vi "PH_Tektronix_7000.PC Write PSDB.vi"(0 "i ref in":refnum<vi>, 5 "error IO":errorcluster) -> (14 "i ref out":refnum<vi>, 19 "error out":errorcluster)   [LabVIEW 2014, in "PH_Tektronix_7000.lvlib"]
doc: "This is the proc case which writes data to the PHELIX shot data base."
uses:
  PH_Tektronix_7000.lvlib
  PH_PSDBWriter/PH_PSDBWriter.String dataset.ctl
  PH_PSDBWriter/PH_PSDBWriter.Numeric dataset.ctl
  PH_StatusHandler/PH_StatusHandler.lvlib
  PH_PSDBWriter/PH_PSDBWriter.lvlib
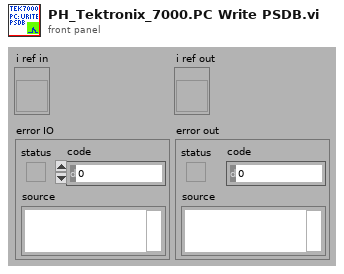
[diagram p1: front panel]
types:
  T1 = typedef "PH_PSDBWriter.lvlib/PH_PSDBWriter.Numeric dataset.ctl" = cluster{"name":string, "data":dbl, "unit":string}
  T2 = typedef "PH_PSDBWriter.lvlib/PH_PSDBWriter.String dataset.ctl" = cluster{"name":string, "data":string, "unit":string}
  T3 = typedef "PH_Tektronix_7000.lvlib/PH_Tektronix_7000.i attribute.ctl" = cluster{"VISA Resource Name":refnum<visa-resource-name>, "IDN":cluster{"Instrument Driver":string, "Instrument Firmware":string, "Model":string, "Serial Number":string}, "Selftest":cluster{"Result":i32, "Message":string}, "Trigger Configuration":T4, "Acquisition Configuration":T5, "GUI Refs":T6, "State":T7, "Error Message":string, "Allow Prdc Loop?":bool, "Channel 1":T8, "Channel 2":T8, "Channel 3":T8, "Channel 4":T8, "Data CH 1":waveform(dbl), "Data CH 2":waveform(dbl), "Data CH 3":waveform(dbl), "Data CH 4":waveform(dbl), "Allow config?":bool, "Name Channel 1":string, "Name Channel 2":string, "Name Channel 3":string, "Name Channel 4":string, "Fetch Data before sending to PSDB?":bool, "Constructor passed?":bool, "Data taken at":timestamp, "Plot Colors":u32[], "Default VISA Resource":string}
  T4 = typedef "PH_Tektronix_7000.lvlib/PH_Tektronix_7000.Trigger Config.ctl" = cluster{"Source":u16, "Level [V]":dbl, "Slope":u16, "Coupling":u16, "Trigger Mode":u16}
  T5 = typedef "PH_Tektronix_7000.lvlib/PH_Tektronix_7000.Acquisition Config.ctl" = cluster{"Record Length":u32, "Timebase [s/div]":dbl, "Position [%]":dbl, "Acquisition Type":u16, "Average Waveforms":i32, "Envelope Waveforms":i32, "WfmDB Samples":i32, "Continuous?":bool, "Delay [s]":dbl, "Run?":bool}
  T6 = typedef "PH_Tektronix_7000.lvlib/PH_Tektronix_7000.GUI Refs.ctl" = cluster{"Graph":refnum<vi>, "State":refnum<vi>, "Delete":refnum<vi>, "VISA Resource":refnum<vi>, "Allow Configure":refnum<vi>, "Fetch Data":refnum<vi>, "Fetch before sending Data to PSDB":refnum<vi>, "Name Channel 1":refnum<vi>, "Name Channel 2":refnum<vi>, "Name Channel 3":refnum<vi>, "Name Channel 4":refnum<vi>, "Prdc Intervall [ms]":refnum<vi>, "Data taken":refnum<vi>, "Model":refnum<vi>, "Serial Number":refnum<vi>, "Firmware":refnum<vi>, "Driver":refnum<vi>, "Acquisition":refnum<vi>, "Trigger":refnum<vi>, "Cursor: D Time [s]":refnum<vi>, "Cursor: D Signal [V]":refnum<vi>, "Channel 1":refnum<vi>, "Channel 2":refnum<vi>, "Channel 3":refnum<vi>, "Channel 4":refnum<vi>}
  T7 = typedef "PH_StatusHandler.lvlib/PH_StatusHandler.Status.ctl" = i16
  T8 = typedef "PH_Tektronix_7000.lvlib/PH_Tektronix_7000.Channel Config.ctl" = cluster{"Enable Channel":bool, "Bandwidth":u16, "Input Impedance":u16, "Vertical Coupling":u16, "Probe Attenuation":dbl, "Range [V/div]":dbl, "Position [div]":dbl, "Bandwidth raw":string}
  T9 = typedef "PH_PSDBWriter.lvlib/PH_PSDBWriter.Boolean dataset.ctl" = cluster{"name":string, "data":bool, "unit":string}
  T10 = typedef "PH_PSDBWriter.lvlib/PH_PSDBWriter.2D dataset.ctl" = cluster{"name":string, "data":dbl[][], "axis description":T11}
  T11 = typedef "PSDB.lvlib/PSDB_AxisDescription.ctl" = cluster{"x axis label":string, "y axis label":string, "x axis unit":string, "y axis unit":string}
  T12 = typedef "PH_PSDBWriter.lvlib/PH_PSDBWriter.PSDB Dataset.ctl" = cluster{"Version":i32, "2D data Input":T10[], "Boolean Input":T9[], "Image Input":T13[], "Numeric Input":T1[], "String Input":T2[]}
  T13 = typedef "PH_PSDBWriter.lvlib/PH_PSDBWriter.Image dataset.ctl" = cluster{"name":string, "data":T14, "unit":string}
  T14 = typedef "IMAQ Image.ctl" = refnum<image>
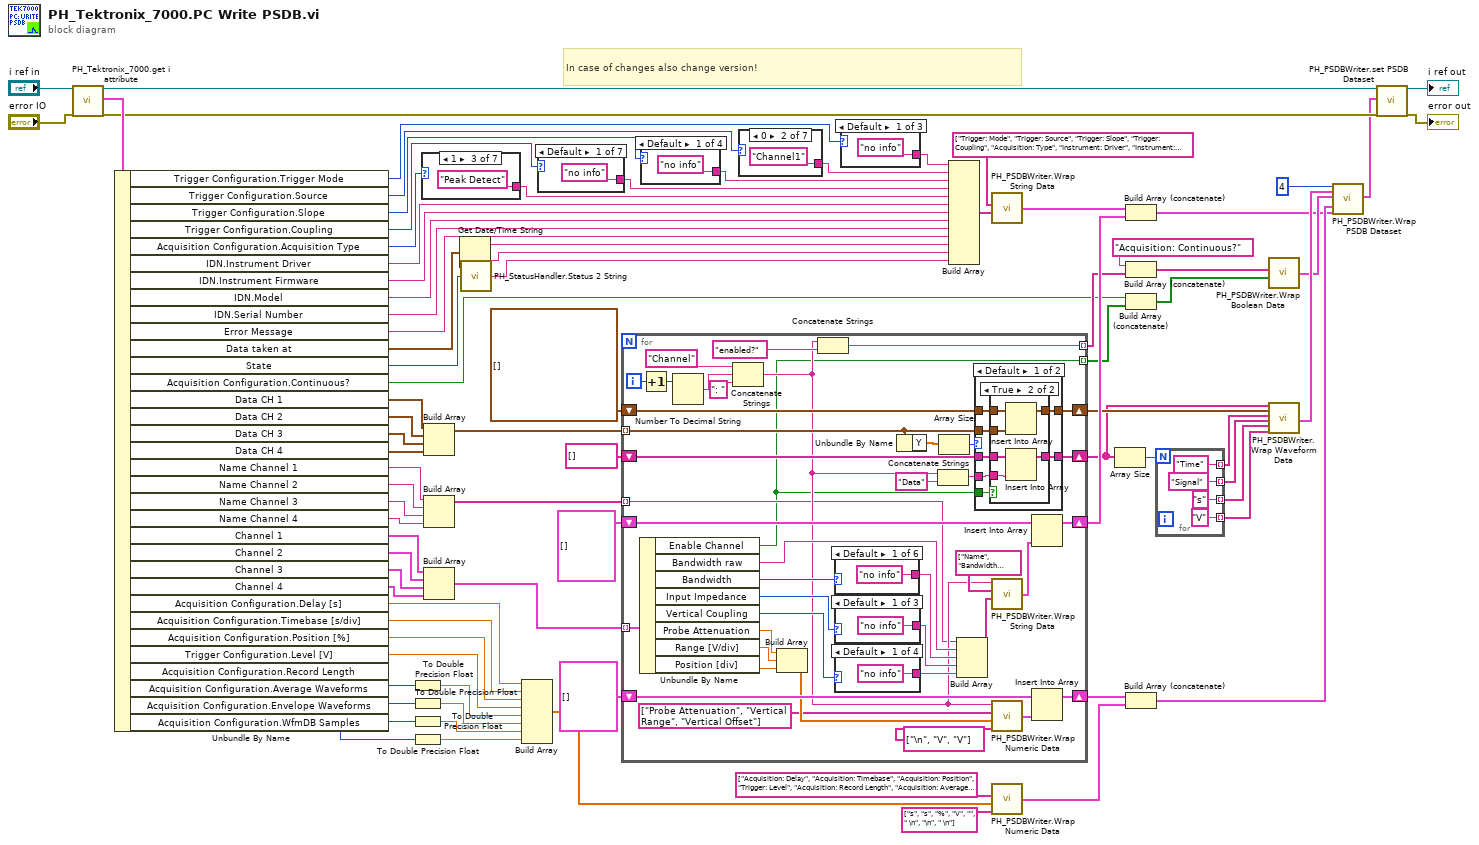
[diagram p0: block diagram]
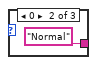
[diagram p2: hidden frame]
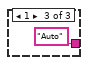
[diagram p3: hidden frame]
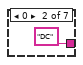
[diagram p4: hidden frame]
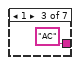
[diagram p5: hidden frame]
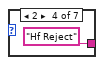
[diagram p6: hidden frame]
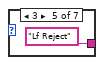
[diagram p7: hidden frame]
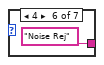
[diagram p8: hidden frame]
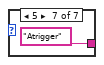
[diagram p9: hidden frame]
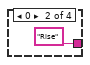
[diagram p10: hidden frame]
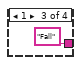
[diagram p11: hidden frame]
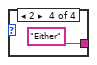
[diagram p12: hidden frame]
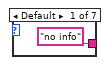
[diagram p13: hidden frame]
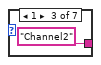
[diagram p14: hidden frame]
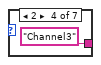
[diagram p15: hidden frame]
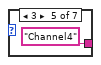
[diagram p16: hidden frame]
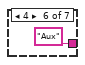
[diagram p17: hidden frame]
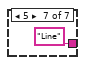
[diagram p18: hidden frame]
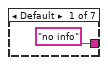
[diagram p19: hidden frame]
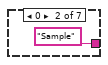
[diagram p20: hidden frame]
diagram:
  # "In case of changes also change version!"
  n1 = call "PH_Tektronix_7000.get i attribute.vi"("i ref in"="i ref in", "error in (no error)"="error IO") -> ("i ref out"=w8:refnum<vi>, "i attribute"=w86:T3, "error out"=w83:errorcluster)  [unwired: 15 in]
  n2 = Unbundle By Name(w86) -> ("Trigger Configuration.Trigger Mode"=w10:u16, "Trigger Configuration.Source"=w23:u16, "Trigger Configuration.Slope"=w13:u16, "Trigger Configuration.Coupling"=w12:u16, "Acquisition Configuration.Acquisition Type"=w19:u16, "IDN.Instrument Driver"=w18:string, "IDN.Instrument Firmware"=w17:string, "IDN.Model"=w16:string, "IDN.Serial Number"=w15:string, "Error Message"=w14:string, "Data taken at"=w74:timestamp, "State"=w76:T7, "Acquisition Configuration.Continuous?"=w26:bool, "Data CH 1"=w82:waveform(dbl), "Data CH 2"=w81:waveform(dbl), "Data CH 3"=w80:waveform(dbl), "Data CH 4"=w79:waveform(dbl), "Name Channel 1"=w61:string, "Name Channel 2"=w62:string, "Name Channel 3"=w63:string, "Name Channel 4"=w25:string, "Channel 1"=w65:T8, "Channel 2"=w66:T8, "Channel 3"=w67:T8, "Channel 4"=w68:T8, "Acquisition Configuration.Delay [s]"=w45:dbl, "Acquisition Configuration.Timebase [s/div]"=w44:dbl, "Acquisition Configuration.Position [%]"=w43:dbl, "Trigger Configuration.Level [V]"=w42:dbl, "Acquisition Configuration.Record Length"=w37:u32, "Acquisition Configuration.Average Waveforms"=w36:i32, "Acquisition Configuration.Envelope Waveforms"=w35:i32, "Acquisition Configuration.WfmDB Samples"=w34:i32)
  n3 = To Double Precision Float(number=w37) -> (double precision float=w33:dbl)
  n4 = To Double Precision Float(number=w36) -> (double precision float=w32:dbl)
  n5 = To Double Precision Float(number=w35) -> (double precision float=w31:dbl)
  n6 = To Double Precision Float(number=w34) -> (double precision float=w30:dbl)
  n7 = case shown="1" w19 {
    tunnel: ["no info" ("string") "Sample" ("string") "Peak Detect" ("string") "Hi Res" ("string") "Average" ("string") "Envelope" ("string") "WfmDB" ("string")] -> w20
    frame Default {
    }
    frame 0 {
    }
    frame 1 {
    }
    frame 2 {
    }
    frame 3 {
    }
    frame 4 {
    }
    frame 5 {
    }
  }
  n8 = Build Array(w82, w81, w80, w79) -> (w78:waveform(dbl)[])
  n9 = Build Array(w61, w62, w63, w25) -> (w29:string[])
  n10 = Build Array(w65, w66, w67, w68) -> (w64:T8[])
  n11 = Get Date/Time String(seconds (now)=w74) -> (date string=w72:string, time string=w73:string)  [unwired: 2 in]
  n12 = call "PH_StatusHandler.Status 2 String.vi"("Status"=w76) -> ("Status as string"=w71:string)
  n13 = Build Array(w45, w44, w43, w42, w33, w32, w31, w30) -> (w41:dbl[])
  n14 = case shown="Default" w12 {
    tunnel: ["no info" ("string") "DC" ("string") "AC" ("string") "Hf Reject" ("string") "Lf Reject" ("string") "Noise Rej" ("string") "Atrigger" ("string")] -> w22
    frame Default {
    }
    frame 0 {
    }
    frame 1 {
    }
    frame 2 {
    }
    frame 3 {
    }
    frame 4 {
    }
    frame 5 {
    }
  }
  n15 = for {
    tunnel: w78 -> [w135] mode=indexing
    tunnel: w29 -> [w102] mode=indexing
    shift-right: [w140] -> w51
    shift-left: string[] [] -> [w139]
    shift-right: [w137] -> w52
    shift-left: waveform(dbl)[] [] -> [w136]
    tunnel: w64 -> [w130] mode=indexing
    shift-right: [w121] -> w59
    shift-left: T2[] [] -> [w113]
    shift-right: [w119] -> w56
    shift-left: T1[] [] ("Tek 7000 PSDB Numeric Data 2") -> [w120]
    tunnel: [w110] -> w28 mode=indexing
    tunnel: [w101] -> w55 mode=indexing
    i -> [w133]
    n16 = Unbundle By Name(w130) -> ("Enable Channel"=w101:bool, "Bandwidth raw"=w105:string, "Bandwidth"=w128:u16, "Input Impedance"=w126:u16, "Vertical Coupling"=w125:u16, "Probe Attenuation"=w114:dbl, "Range [V/div]"=w115:dbl, "Position [div]"=w116:dbl)
    n17 = Increment(x=w133) -> (x+1=w132:i32)
    n18 = Number To Decimal String(number=w132) -> (decimal integer string=w131:string)  [unwired: 1 in]
    n19 = Concatenate Strings("Channel", w131, ": " ("string")) -> (w103:string)
    n20 = Build Array(w114, w115, w116) -> (w108:dbl[])
    n21 = Concatenate Strings(w103, "enabled?" ("string")) -> (w110:string)
    n22 = case shown="Default" w128 {
      tunnel: ["no info" ("string") "FULL" ("string") "500 MHz" ("string") "250 MHz" ("string") "150 MHz" ("string") "20 MHz" ("string")] -> w124
      frame Default {
      }
      frame 0 {
      }
      frame 1 {
      }
      frame 2 {
      }
      frame 3 {
      }
      frame 4 {
      }
    }
    n23 = case shown="Default" w126 {
      tunnel: ["no info" ("string") "1M" ("string") "50" ("string")] -> w123
      frame Default {
      }
      frame 0 {
      }
      frame 1 {
      }
    }
    n24 = case shown="Default" w125 {
      tunnel: ["no info" ("string") "AC" ("string") "DC" ("string") "Ground" ("string")] -> w122
      frame Default {
      }
      frame 0 {
      }
      frame 1 {
      }
      frame 2 {
      }
    }
    n25 = Unbundle By Name(w135) -> ("Y"=w138:dbl[])
    n26 = Concatenate Strings(w103, "Data" ("string")) -> (w129:string)
    n27 = Array Size(array=w138) -> (size(s)=w141:i32)
    n28 = Build Array(w102, w105, w124, w123, w122) -> (w111:string[])
    n29 = case shown="Default" w141 {
      tunnel: w129 -> [w161 _]
      tunnel: [w160 w171] -> w140
      tunnel: w139 -> [w159 w171]
      tunnel: [w158 w170] -> w137
      tunnel: w136 -> [w157 w170]
      tunnel: w135 -> [w156 _]
      tunnel: w101 -> [w155 _]
      frame Default {
        n30 = case shown="True" w155 {
          tunnel: w161 -> [_ w169]
          tunnel: [w163 w168] -> w160
          tunnel: w159 -> [w163 w167]
          tunnel: [w162 w166] -> w158
          tunnel: w157 -> [w162 w165]
          tunnel: w156 -> [_ w164]
          frame False {
          }
          frame True {
            n31 = Insert Into Array(array=w165, new element=w164) -> (w166:waveform(dbl)[])  [unwired: 1 in]
            n32 = Insert Into Array(array=w167, new element=w169) -> (w168:string[])  [unwired: 1 in]
          }
        }
      }
      frame 0 {
      }
    }
    n33 = call "PH_PSDBWriter.Wrap String Data.vi"("Data Array"=w111, "Name Array"=string[] ["Name", "Bandwidth (raw)", "Bandwidth", "Impedance", "Coupling"], "Name Prefix"=w103) -> ("PSDB String Data Array"=w112:T2[])  [unwired: 1 in]
    n34 = call "PH_PSDBWriter.Wrap Numeric Data.vi"("Unit Array"=string[] ["\n", "V", "V"], "Data Array"=w108, "Name Array"=string[] ["Probe Attenuation", "Vertical Range", "Vertical Offset"], "Name Prefix"=w103) -> ("PSDB Numeric Data Array"=w118:T1[])
    n35 = Insert Into Array(array=w113, new element=w112) -> (w121:T2[])  [unwired: 1 in]
    n36 = Insert Into Array(array=w120, new element=w118) -> (w119:T1[])  [unwired: 1 in]
  }
  n37 = case shown="Default" w13 {
    tunnel: ["no info" ("string") "Rise" ("string") "Fall" ("string") "Either" ("string")] -> w21
    frame Default {
    }
    frame 0 {
    }
    frame 1 {
    }
    frame 2 {
    }
  }
  n38 = case shown="0" w23 {
    tunnel: ["no info" ("string") "Channel1" ("string") "Channel2" ("string") "Channel3" ("string") "Channel4" ("string") "Aux" ("string") "Line" ("string")] -> w24
    frame Default {
    }
    frame 0 {
    }
    frame 1 {
    }
    frame 2 {
    }
    frame 3 {
    }
    frame 4 {
    }
    frame 5 {
    }
  }
  n39 = case shown="Default" w10 {
    tunnel: ["no info" ("string") "Normal" ("string") "Auto" ("string")] -> w11
    frame Default {
    }
    frame 0 {
    }
    frame 1 {
    }
  }
  n40 = Build Array(w11, w24, w21, w22, w20, w18, w17, w16, w15, w14, w72, w73, w71) -> (w70:string[])
  n41 = call "PH_PSDBWriter.Wrap String Data.vi"("Data Array"=w70, "Name Array"=string[] ["Trigger: Mode", "Trigger: Source", "Trigger: Slope", "Trigger: Coupling", "Acquisition: Type", "Instrument: Driver", "Instrument: Firmware", "Instrument: Model", "Instrument: Serial Number", "Instrument: Error Message", "Data taken on", "Data taken at", "Device Status"]) -> ("PSDB String Data Array"=w60:T2[])  [unwired: 2 in]
  n42 = call "PH_PSDBWriter.Wrap Numeric Data.vi"("Unit Array"=string[] ["s", "s", "%", "V", "", " \n", "\n", " \n"], "Data Array"=w41, "Name Array"=string[] ["Acquisition: Delay", "Acquisition: Timebase", "Acquisition: Position", "Trigger: Level", "Acquisition: Record Length", "Acquisition: Average Waveforms", "Acquisition: Envelope Waveforms", "Acquisition: WfmDB Samples"]) -> ("PSDB Numeric Data Array"=w40:T1[])  [unwired: 1 in]
  n43 = Array Size(array=w51) -> (size(s)=w50:i32)
  n44 = Build Array (concatenate)(w60, w59) -> (w2:T2[])
  n45 = Build Array (concatenate)("Acquisition: Continuous?" ("name"), w28) -> (w54:string[])
  n46 = Build Array (concatenate)(w26, w55) -> (w53:bool[])
  n47 = Build Array (concatenate)(w56, w40) -> (w3:T1[])
  n48 = for {
    N: w50 -> [_]
    tunnel: ["Time" ("x axis label")] -> w49 mode=indexing
    tunnel: ["Signal" ("y axis label")] -> w48 mode=indexing
    tunnel: ["s" ("x axis unit")] -> w47 mode=indexing
    tunnel: ["V" ("y axis unit")] -> w46 mode=indexing
  }
  n49 = call "PH_PSDBWriter.Wrap Boolean Data.vi"("Data Array"=w53, "Name Array"=w54) -> ("PSDB Boolean Data Array"=w4:T9[])  [unwired: 2 in]
  n50 = call "PH_PSDBWriter.Wrap Waveform Data.vi"("Name Array"=w51, "Data Array"=w52, "x axis label Array"=w49, "y axis label Array"=w48, "x axis unit Array"=w47, "y axis unit Array"=w46) -> ("PSDB 2D Data Array"=w5:T10[])  [unwired: 13 in]
  n51 = call "PH_PSDBWriter.Wrap PSDB Dataset.vi"("Version"=4, "2D data Input"=w5, "Boolean Input"=w4, "Numeric Input"=w3, "String Input"=w2) -> ("PSDB Dataset"=w6:T12)  [unwired: 14 in]
  n52 = call "PH_PSDBWriter.set PSDB Dataset.vi"("VI in"=w8, "PSDB Dataset"=w6, "error in (no error)"=w83) -> ("VI out"=→"i ref out":refnum<vi>, "error out"=→"error out":errorcluster)  [unwired: 15 in]
